vi "EdgeTool(subVI).vi"(6 "error in (no error)":errorcluster, 9 "New Image":T1) -> (0 "error out":errorcluster, 2 "Edge Information":T2[](array[typedef]) {"Distance (Real-World)" format="%.2f"; "Location (Real-World)"."Y" format="%.2g"; "Location (Real-World)"."X" format="%.2f"; "Noise" format="%.2f"; "Location (Pixel)"."Y" format="%.2g"; "Location (Pixel)"."X" format="%.2f"; "Strength" format="%.2f"; "Distance (Pixel)" format="%.2f"}, 3 "Image Out":T1)   [LabVIEW 2020]
doc: "Verifica che il numero degli Edge sia uguale a quello indicato nel campo \"numero\"."
uses:
  <vilib>/vision/Measure.llb/Edge Options.ctl
  <vilib>/vision/Measure.llb/Edge Polarity.ctl
  <vilib>/vision/Measure.llb/Edge New.ctl
  <vilib>/vision/Image Controls.llb/IMAQ Image.ctl
  <vilib>/vision/NI_Vision_Development_Module.lvlib
panel:
  in  "Stop":bool
  in  "Edge Options":T3={"Edge Polarity"=0, "Kernel Size"=3, "Width"=3, "Minimum Edge Strength"=10.0, "Interpolation Type"=enum."Bilinear Fixed", "Data Processing Method"=enum."Average"} {"Edge Polarity" items=["All Edges", "Rising Edges", "Falling Edges"]; "Minimum Edge Strength" format="%.2f"; "Width" step=2; "Kernel Size" step=2}
  out "Gradient Information":dbl[](graph)
  out "Image":T1(plugin-control)
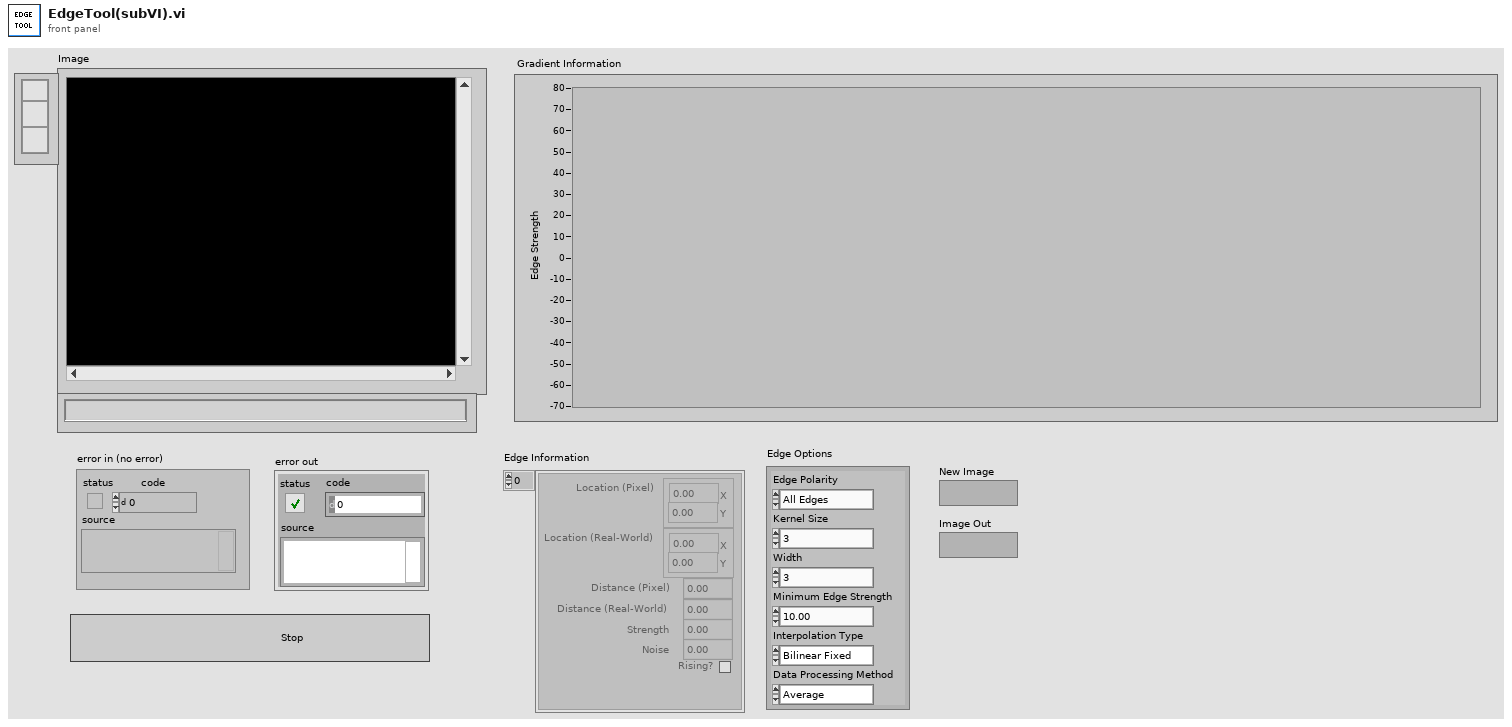
[diagram p1: front panel]
types:
  T1 = typedef "IMAQ Image.ctl" = refnum<image>
  T2 = typedef "Edge New.ctl" = cluster{"Location (Pixel)":cluster{"X":sgl, "Y":sgl}, "Location (Real-World)":cluster{"X":sgl, "Y":sgl}, "Distance (Pixel)":dbl, "Distance (Real-World)":dbl, "Strength":dbl, "Noise":dbl, "Rising?":bool}
  T3 = typedef "Edge Options.ctl" = cluster{"Edge Polarity":T4, "Kernel Size":u32, "Width":u32, "Minimum Edge Strength":sgl, "Interpolation Type":enum32{"Zero Order", "Bilinear", "Quadratic", "Cubic", "Bilinear Fixed"}, "Data Processing Method":enum32{"Average", "Median"}}
  T4 = typedef "Edge Polarity.ctl" = u32
  T5 = typedef "IMAQ Line" = cluster{"Start X":i32, "Start Y":i32, "End X":i32, "End Y":i32}
  T6 = typedef "ROI Descriptor" = cluster{"Global Rectangle":i32[], "Contours":cluster{"ID":enum32{"External", "Internal"}, "Type":u32, "Coordinates":i32[]}[]}
  T7 = cluster{"Global Rectangle":i32[], "Contours":cluster{"Contour Type":u32, "ROI Type":u32, "Points":i32[]}[]}
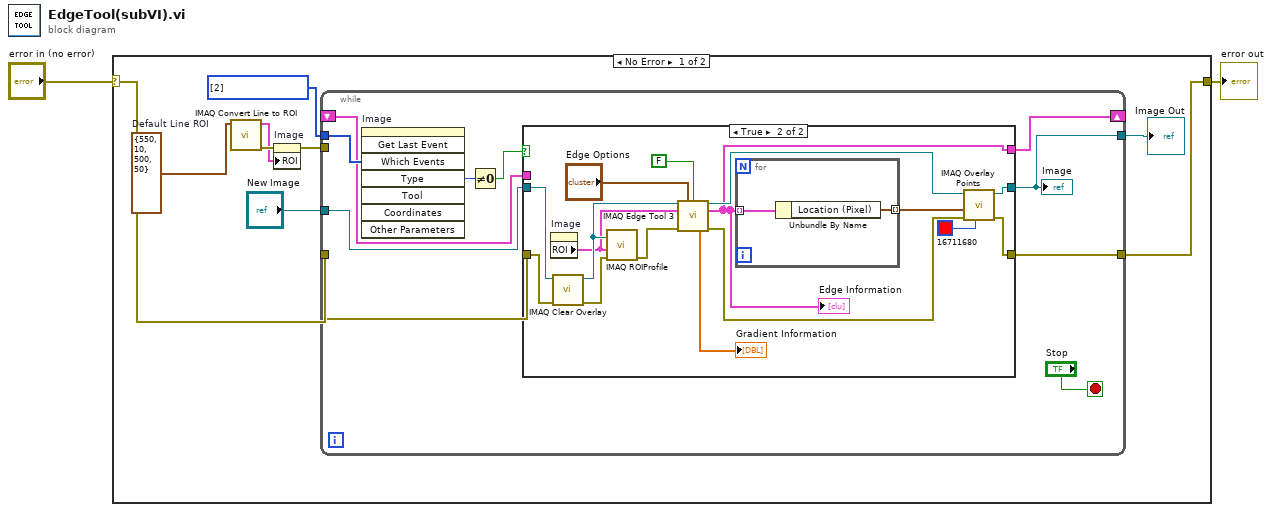
[diagram p0: block diagram]
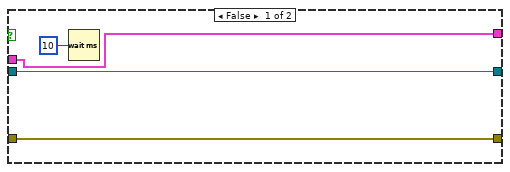
[diagram p2: hidden frame]
diagram:
  n1 = case shown="No Error" "error in (no error)" {
    selector: "error in (no error)" -> [w4 w44]
    tunnel: [w5 w44] -> w2
    frame No Error {
      w10 = T5 {"Start X"=550, "Start Y"=10, "End X"=500, "End Y"=50}  # Default Line ROI
      w11 = i32[] [2] items=["No  event", "Click event", "Draw event", "Move event", "Size event", "Scroll event", "Activate event", "Close event", "Double click event"] ("Events list (all)")
      n2 = call "IMAQ Convert Line to ROI"("Line"=w10) -> ("error out"=w9:errorcluster, "ROI Descriptor"=w8:T6)  [unwired: 8 in]
      n3 = property on="Image" class="ImageControl"(error in=w9, "ROI"=w8) -> (error out=w7:errorcluster)  [unwired: 1 in, 1 out]
      n4 = while {
        tunnel: "New Image" -> [w17]
        tunnel: [w21] -> w5
        tunnel: w11 -> [w20]
        tunnel: w7 -> [_]
        tunnel: w4 -> [w15]
        shift-right: [w14] -> _
        shift-left: _ -> [w13]
        tunnel: [w12] -> w3
        stop <- "Stop" stop-if-true
        n5 = invoke on="Image" class="ImageControl" method="Get Last Event"("Which Events"=w20) -> ("Type"=w19:i32)  [unwired: 7 in, 7 out]
        n6 = Not Equal To 0?(x=w19) -> (x != 0?=w18:bool)
        n7 = case shown="True" w18 {
          tunnel: w17 -> [w25 w40]
          tunnel: [w25 w29] -> w12
          tunnel: [w23 w30] -> w21
          tunnel: w15 -> [w23 w27]
          tunnel: [w22 w26] -> w14
          tunnel: w13 -> [w22 _]
          frame False {
            n8 = Wait (ms)(milliseconds to wait=u32 10) -> ()  [unwired: 1 out]
          }
          frame True {
            n9 = property on="Image" class="ImageControl"() -> ("ROI"=w36:T7)  [unwired: 2 in, 2 out]
            n10 = call "IMAQ Clear Overlay"("error in (no error)"=w27, "Image"=w40) -> ("error out"=w38:errorcluster, "Image Out"=w39:T1)  [unwired: 8 in]
            n11 = call "IMAQ ROIProfile"("error in (no error)"=w38, "ROI Descriptor"=w36, "Image"=w39) -> ("error out"=w41:errorcluster)  [unwired: 1 in, 4 out]
            n12 = call "IMAQ Edge Tool 3"("Image"=w39, "Edge Options"="Edge Options", "Optimized Mode"=FALSE, "ROI Descriptor"=w36, "error in (no error)"=w41) -> ("Image (duplicate)"=w33:T1, "Edge Information"=w26:T2[], "Gradient Values"=→"Gradient Information":dbl[], "error out"=w31:errorcluster)  [unwired: 6 in, 1 out]
            "Edge Information" <- w26
            n13 = for {
              tunnel: w26 -> [w43] mode=indexing
              tunnel: [w42] -> w32 mode=indexing
              n14 = Unbundle By Name(w43) -> ("Location (Pixel)"=w42:cluster{"X":sgl, "Y":sgl})
            }
            n15 = call "IMAQ Overlay Points"("Color"=u32 16711680, "error in (no error)"=w31, "Array of Points"=w32, "Image"=w33) -> ("error out"=w30:errorcluster, "Image Out"=w29:T1)  [unwired: 6 in]
          }
        }
        "Image" <- w12
      }
      "Image Out" <- w3
    }
    frame Error {
    }
  }
  "error out" <- w2
